vi "JGE1.vi"() -> ()   [LabVIEW 2019]
doc: "Exercise 1 this vi Uses a manuel input signal or an automatic signel and then applies a high pass filter to the signal \n\nJuan Gamez\nP3600\nCSUSB"
uses:
  typedefs/source control type.ctl
panel:
  out "Auto ON":bool
  in  "source controls":T1={"signal choice"=FALSE, "amplitude"=1.0, "period"=50.0, "reset source"=FALSE} {"period" scale=1.0..1000.0; "amplitude" scale=0.0..2.0}
  in  "AutoGenerate signal":bool
  in  "Corner period":dbl(slide)=30.0 scale=1.0..1000.0
  in  "Manual Input +1 or -1":bool
  in  "stop":bool
  out "Signal Monitor":cluster{"output":dbl, "output":dbl}(graph)={"output"=-0.48175367410171677, "output"=0.14037848618672943}
  # "High Pass Filter"
  # "Flow Control"
  # "Juan Gamez\nP3600\nCSUSB"
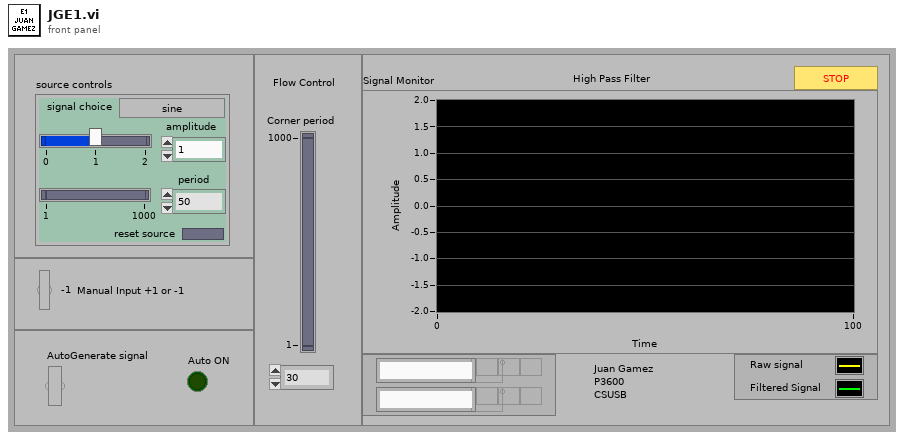
[diagram p1: front panel]
types:
  T1 = typedef "source control type.ctl" = cluster{"signal choice":bool, "amplitude":dbl, "period":dbl, "reset source":bool}
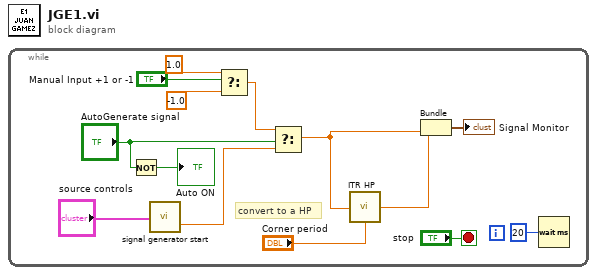
[diagram p0: block diagram]
diagram:
  n1 = while {
    stop <- "stop" stop-if-true
    # "convert to a HP"
    n2 = Not(x="AutoGenerate signal") -> (.not. x?=→"Auto ON":bool)
    n3 = call "signal generator start.vi"("source controls"="source controls") -> ("signal output"=w3:dbl)  [unwired: 14 in]
    n4 = Select(t=1.0, s="Manual Input +1 or -1", f=-1.0) -> (s? t:f=w6:dbl)
    n5 = Select(t=w6, s="AutoGenerate signal", f=w3) -> (s? t:f=w5:dbl)
    n6 = call "ITR HP.vi"("input"=w5, "corner period (steps)"="Corner period") -> ("output"=w12:dbl)  [unwired: 13 in]
    n7 = Bundle("signal output"=w5, "output"=w12) -> (→"Signal Monitor":cluster{"signal output":dbl, "output":dbl})  [unwired: 1 in]
    n8 = Wait (ms)(milliseconds to wait=u32 20 ("solution S12")) -> ()  [unwired: 1 out]
  }
